vi "Dataset Source 2 Volt Types.vi"(10 "Dataset Source":T2=enum."External Sensors") -> (1 "No Volt Types Out":T1[](array[typedef]), 2 "Volt Types":T1[](array[typedef])=[enum."LVDT"])   [LabVIEW 2009]
uses:
  Dataset Source.ctl
  Dataset Type.ctl
panel:
  in  "Volt Types":T1[](array[typedef])=[enum."Actuator Command", enum."LVDT", enum."Load Cell", enum."Servo Error"]
  in  "External Sensor Types":T1[](array[typedef])=[enum."LVDT"]
  in  "Non Volt Types":T1[](array[typedef])=[enum."Displacement Command", enum."Displacement", enum."Force"]
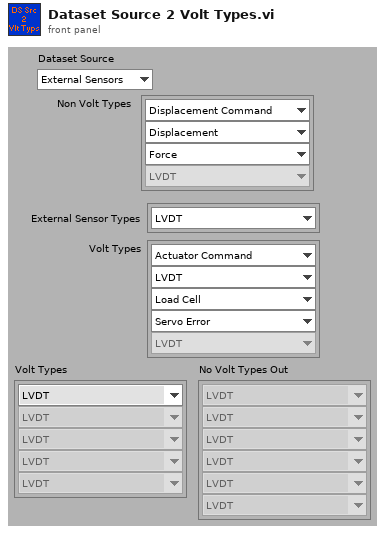
[diagram p1: front panel]
types:
  T1 = typedef "Dataset Type.ctl" = enum16{"LVDT", "Load Cell", "Actuator Command", "Servo Error", "Displacement Command", "Displacement", "Force"}
  T2 = typedef "Dataset Source.ctl" = enum16{"LBCB 1", "LBCB 2", "Combined", "External Sensors"}
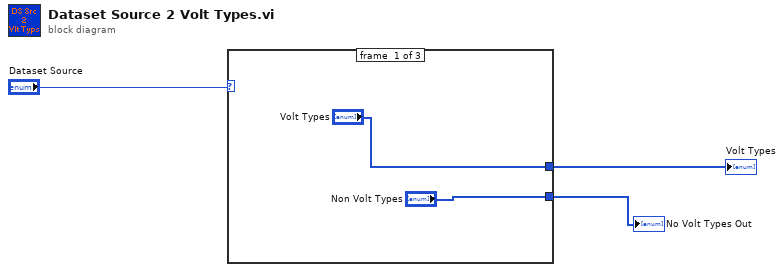
[diagram p0: block diagram]
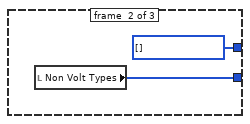
[diagram p2: hidden frame]
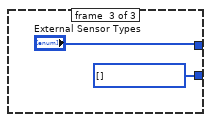
[diagram p3: hidden frame]
diagram:
  n1 = case shown="\"Combined\"" "Dataset Source" {
    tunnel: ["Volt Types" w7 "External Sensor Types"] -> w2
    tunnel: ["Non Volt Types" w6 w8] -> w1
    frame #0 {
    }
    frame #1 {
      w7 = T1[] [] items=["LVDT", "Load Cell", "Actuator Command", "Servo Error", "Displacement Command", "Displacement", "Force"] ("External Sensor Types")
      n2 = local read "Non Volt Types"() -> (w6:T1[])
    }
    frame #2 {
      w8 = T1[] [] items=["LVDT", "Load Cell", "Actuator Command", "Servo Error", "Displacement Command", "Displacement", "Force"] ("Combined Types")
    }
  }
  "Volt Types" <- w2
  "No Volt Types Out" <- w1
